vi "_scriptEditor CSM State Selection.vi"(9 "Pos":i32, 11 "single-line text":string) -> (0 "Msg Type":T3=enum."Message", 2 "Selection":T2, 3 "Selection 2":cluster{"end":i32, "start":i32})   [LabVIEW 2017]
uses:
  def-message type.ctl
  def-Selection Type.ctl
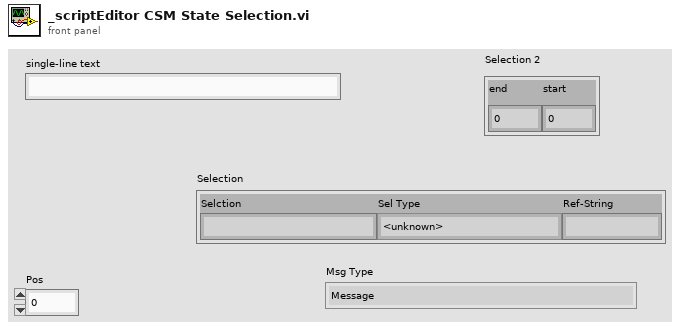
[diagram p1: front panel]
types:
  T1 = typedef "def-Selection Type.ctl" = enum16{"<unknown>", "Reg-Oper", "Reg-Symbol", "Msg-State", "Msg-Arg", "Msg-ArgSymbol", "Msg-Symbol", "Comments", "Broadcast-Symbol", "Broadcasst-Oper"}
  T2 = cluster{"Selction":string, "Sel Type":T1, "Ref-String":string}
  T3 = typedef "def-message type.ctl" = enum16{"State", "Message", "Broadcast", "Registration"}
  T4 = cluster{"single-line text":string, T1, "Ref-String":string}
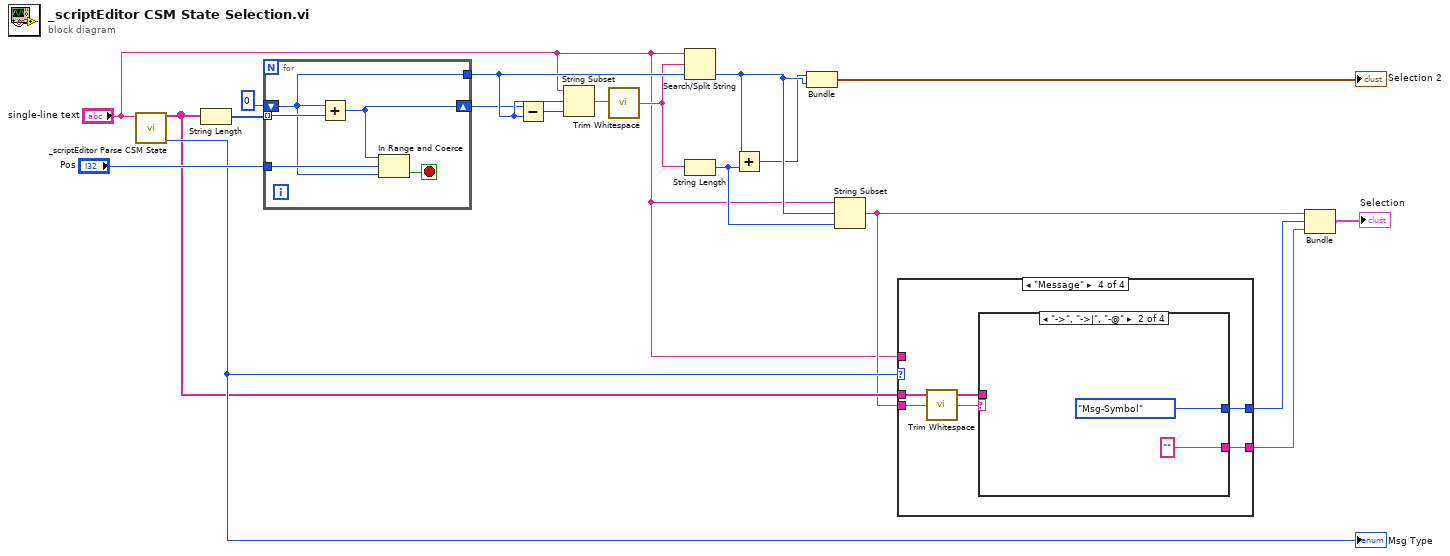
[diagram p0: block diagram]
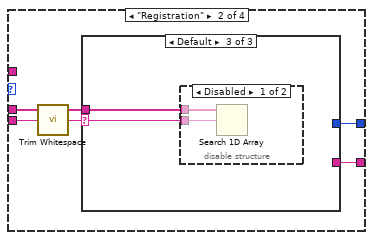
[diagram p3: hidden frame]
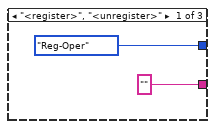
[diagram p4: hidden frame]
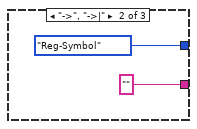
[diagram p5: hidden frame]
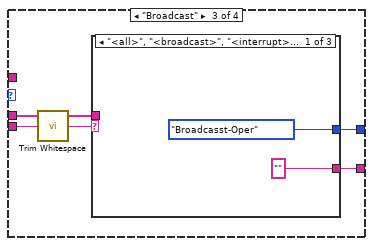
[diagram p7: hidden frame]
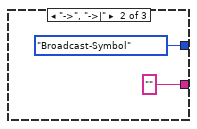
[diagram p8: hidden frame]
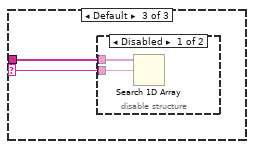
[diagram p9: hidden frame]
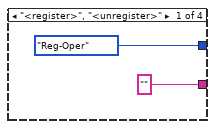
[diagram p11: hidden frame]
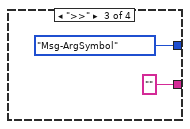
[diagram p12: hidden frame]
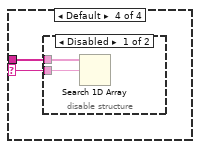
[diagram p13: hidden frame]
diagram:
  n1 = call "_scriptEditor Parse CSM State.vi"("single-line text"="single-line text") -> ("Msg Type"=w9:T3, "Array"=w8:string[])  [unwired: 9 in]
  "Msg Type" <- w9
  n2 = String Length(string=w8) -> (length=w17:i32[])
  n3 = for {
    tunnel: w17 -> [w23] mode=indexing
    tunnel: "Pos" -> [w24]
    shift-right: [w21] -> w12
    shift-left: 0 ("element") -> [w20]
    tunnel: [w20] -> w14
    stop <- w22 stop-if-true
    n4 = Add(x=w20, y=w23) -> (x+y=w21:i32)
    n5 = In Range and Coerce(upper limit=w21, x=w24, lower limit=w20) -> (In Range?=w22:bool)  [unwired: 1 out]
  }
  n6 = Subtract(x=w12, y=w14) -> (x-y=w16:i32)
  n7 = String Subset(string="single-line text", offset (0)=w14, length (rest)=w16) -> (substring=w15:string)
  n8 = call <vilib>:"Trim Whitespace.vi"("string"=w15) -> ("trimmed string"=w13:string)  [unwired: 1 in]
  n9 = Search/Split String(string="single-line text", search string/char (-)=w13, offset (0)=w14) -> (offset of match=w3:i32)  [unwired: 2 out]
  n10 = String Length(string=w13) -> (length=w10:i32)
  n11 = Add(x=w3, y=w10) -> (x+y=w2:i32)
  n12 = Bundle(w2, "offset of match"=w3) -> (→"Selection 2":cluster{i32, "offset of match":i32})  [unwired: 1 in]
  n13 = String Subset(string="single-line text", offset (0)=w3, length (rest)=w10) -> (substring=w7:string)
  n14 = case shown="\"Message\"" w9 {
    tunnel: w8 -> [_ w29 w42 w55]
    tunnel: w7 -> [_ w28 w41 w54]
    tunnel: [_ w27 w40 w53] -> w6
    tunnel: [_ w26 w39 w52] -> w5
    tunnel: "single-line text" -> [_ _ _ _]
    frame "State", Default {
    }
    frame "Registration" {
      n15 = call <vilib>:"Trim Whitespace.vi"("string"=w28) -> ("trimmed string"=w25:string)  [unwired: 1 in]
      n16 = case shown="Default" w25 {
        selector: w25 -> [_ _ w34]
        tunnel: w29 -> [_ _ w35]
        tunnel: [def-Selection_Type."Reg-Oper" def-Selection_Type."Reg-Symbol" _] -> w27
        tunnel: ["" ("Ref-String") "" ("Ref-String") _] -> w26
        frame "<register>", "<unregister>" {
        }
        frame "->", "->|" {
        }
        frame Default {
          n17 = disable-structure shown="Disabled" {
            disable-tunnel: w35 -> [w37 _]
            disable-tunnel: w34 -> [w36 _]
            frame Disabled {
              n18 = Search 1D Array(1D array=w37, element=w36) -> ()  [unwired: 1 in, 1 out]
            }
            frame Enabled {
            }
          }
        }
      }
    }
    frame "Broadcast" {
      n19 = call <vilib>:"Trim Whitespace.vi"("string"=w41) -> ("trimmed string"=w38:string)  [unwired: 1 in]
      n20 = case shown="\"<all>\", \"<broadcast>\", \"<interrupt>\", \"<status>\"" w38 {
        selector: w38 -> [_ _ w47]
        tunnel: w42 -> [_ _ w48]
        tunnel: [def-Selection_Type."Broadcasst-Oper" def-Selection_Type."Broadcast-Symbol" _] -> w40
        tunnel: ["" ("Ref-String") "" ("Ref-String") _] -> w39
        frame "<all>", "<broadcast>", "<interrupt>", "<status>" {
        }
        frame "->", "->|" {
        }
        frame Default {
          n21 = disable-structure shown="Disabled" {
            disable-tunnel: w48 -> [w50 _]
            disable-tunnel: w47 -> [w49 _]
            frame Disabled {
              n22 = Search 1D Array(1D array=w50, element=w49) -> ()  [unwired: 1 in, 1 out]
            }
            frame Enabled {
            }
          }
        }
      }
    }
    frame "Message" {
      n23 = call <vilib>:"Trim Whitespace.vi"("string"=w54) -> ("trimmed string"=w51:string)  [unwired: 1 in]
      n24 = case shown="\"->\", \"->|\", \"-@\"" w51 {
        selector: w51 -> [_ _ _ w62]
        tunnel: w55 -> [_ _ _ w63]
        tunnel: [def-Selection_Type."Reg-Oper" def-Selection_Type."Msg-Symbol" def-Selection_Type."Msg-ArgSymbol" _] -> w53
        tunnel: ["" ("Ref-String") "" ("Ref-String") "" ("Ref-String") _] -> w52
        frame "<register>", "<unregister>" {
        }
        frame "->", "->|", "-@" {
        }
        frame ">>" {
        }
        frame Default {
          n25 = disable-structure shown="Disabled" {
            disable-tunnel: w63 -> [w65 _]
            disable-tunnel: w62 -> [w64 _]
            frame Disabled {
              n26 = Search 1D Array(1D array=w65, element=w64) -> ()  [unwired: 1 in, 1 out]
            }
            frame Enabled {
            }
          }
        }
      }
    }
  }
  n27 = Bundle("single-line text"=w7, w6, "Ref-String"=w5) -> (→"Selection":T4)  [unwired: 1 in]
